vi "Methods_Insert Dividers.vi"(11 "Methods[] In":T1(array[cluster])) -> (3 "Methods[] Out":T1(array[cluster]))   [LabVIEW 2023] (continued)
Symbols:Set To Custom Symbol"}, "Method Flags"={"IsDeprecated"=FALSE, "IsPrivate"=FALSE, "IsScripting"=FALSE, "IsNotInRun-Time"=FALSE}, "Divider"=FALSE}, {"Class Info"={"Unique ID string"="66", "Parent ID string"="6", "Class Name (unlocalized)"="TreeControl", "Class Name (localized)"="TreeControl"}, "Method Info"={"Unique ID string"="756a3812", "Data name"="Custom Item Symbols.Set Symbol Array", "Short name (localized)"="Custom Item Symbols.Set Symbol Array", "Long name (localized)"="Custom Item Symbols:Set To Custom Symbol Array"}, "Method Flags"={"IsDeprecated"=FALSE, "IsPrivate"=FALSE, "IsScripting"=FALSE, "IsNotInRun-Time"=FALSE}, "Divider"=FALSE}, {"Class Info"={"Unique ID string"="66", "Parent ID string"="6", "Class Name (unlocalized)"="TreeControl", "Class Name (localized)"="TreeControl"}, "Method Info"={"Unique ID string"="756a3813", "Data name"="Custom Item Symbols.Revert Symbol", "Short name (localized)"="Custom Item Symbols.Revert Symbol", "Long name (localized)"="Custom Item Symbols:Revert To Built In Symbol"}, "Method Flags"={"IsDeprecated"=FALSE, "IsPrivate"=FALSE, "IsScripting"=FALSE, "IsNotInRun-Time"=FALSE}, "Divider"=FALSE}, {"Class Info"={"Unique ID string"="66", "Parent ID string"="6", "Class Name (unlocalized)"="TreeControl", "Class Name (localized)"="TreeControl"}, "Method Info"={"Unique ID string"="756a3814", "Data name"="Custom Item Symbols.Revert Symbols", "Short name (localized)"="Custom Item Symbols.Revert Symbols", "Long name (localized)"="Custom Item Symbols:Revert All To Built In Symbols"}, "Method Flags"={"IsDeprecated"=FALSE, "IsPrivate"=FALSE, "IsScripting"=FALSE, "IsNotInRun-Time"=FALSE}, "Divider"=FALSE}, {"Class Info"={"Unique ID string"="66", "Parent ID string"="6", "Class Name (unlocalized)"="TreeControl", "Class Name (localized)"="TreeControl"}, "Method Info"={"Unique ID string"="756a3815", "Data name"="Point To Row Column", "Short name (localized)"="Point To Row Column", "Long name (localized)"="Point to Row Column"}, "Method Flags"={"IsDeprecated"=FALSE, "IsPrivate"=FALSE, "IsScripting"=FALSE, "IsNotInRun-Time"=FALSE}, "Divider"=FALSE}, {"Class Info"={"Unique ID string"="66", "Parent ID string"="6", "Class Name (unlocalized)"="TreeControl", "Class Name (localized)"="TreeControl"}, "Method Info"={"Unique ID string"="756a3816", "Data name"="Navigate Tree.Get Previous", "Short name (localized)"="Navigate Tree.Get Previous", "Long name (localized)"="Navigate Tree:Get Previous Item"}, "Method Flags"={"IsDeprecated"=FALSE, "IsPrivate"=FALSE, "IsScripting"=FALSE, "IsNotInRun-Time"=FALSE}, "Divider"=FALSE}, {"Class Info"={"Unique ID string"="66", "Parent ID string"="6", "Class Name (unlocalized)"="TreeControl", "Class Name (localized)"="TreeControl"}, "Method Info"={"Unique ID string"="756a3817", "Data name"="Edit Tree Items.Add Multiple Items to End", "Short name (localized)"="Edit Tree Items.Add Multiple Items to End", "Long name (localized)"="Edit Tree Items:Add Multiple Items to End"}, "Method Flags"={"IsDeprecated"=FALSE, "IsPrivate"=FALSE, "IsScripting"=FALSE, "IsNotInRun-Time"=FALSE}, "Divider"=FALSE}, {"Class Info"={"Unique ID string"="71", "Parent ID string"="6", "Class Name (unlocalized)"="PlugInDDODummyContainer", "Class Name (localized)"="PlugInDDODummyContainer"}, "Method Info"={"Unique ID string"="47813c00", "Data name"="Dummy", "Short name (localized)"="Dummy", "Long name (localized)"="Dummy"}, "Method Flags"={"IsDeprecated"=FALSE, "IsPrivate"=TRUE, "IsScripting"=FALSE, "IsNotInRun-Time"=FALSE}, "Divider"=FALSE}, {"Class Info"={"Unique ID string"="73", "Parent ID string"="", "Class Name (unlocalized)"="Project", "Class Name (localized)"="Project"}, "Method Info"={"Unique ID string"="27109002", "Data name"="Close", "Short name (localized)"="Close", "Long name (localized)"="Close"}, "Method Flags"={"IsDeprecated"=FALSE, "IsPrivate"=FALSE, "IsScripting"=FALSE, "IsNotInRun-Time"=FALSE}, "Divider"=FALSE}, {"Class Info"={"Unique ID string"="73", "Parent ID string"="", "Class Name (unlocalized)"="Project", "Class Name (localized)"="Project"}, "Method Info"={"Unique ID string"="27109003", "Data name"="Save", "Short name (localized)"="Save", "Long name (localized)"="Save"}, "Method Flags"={"IsDeprecated"=FALSE, "IsPrivate"=FALSE, "IsScripting"=FALSE, "IsNotInRun-Time"=TRUE}, "Divider"=FALSE}, {"Class Info"={"Unique ID string"="73", "Parent ID string"="", "Class Name (unlocalized)"="Project", "Class Name (localized)"="Project"}, "Method Info"={"Unique ID string"="27109006", "Data name"="Item From Item ID", "Short name (localized)"="Item From Item ID", "Long name (localized)"="Item From Item ID"}, "Method Flags"={"IsDeprecated"=FALSE, "IsPrivate"=TRUE, "IsScripting"=FALSE, "IsNotInRun-Time"=TRUE}, "Divider"=FALSE}, {"Class Info"={"Unique ID string"="73", "Parent ID string"="", "Class Name (unlocalized)"="Project", "Class Name (localized)"="Project"}, "Method Info"={"Unique ID string"="27109009", "Data name"="Open Window", "Short name (localized)"="Open Window", "Long name (localized)"="Open Window"}, "Method Flags"={"IsDeprecated"=FALSE, "IsPrivate"=FALSE, "IsScripting"=FALSE, "IsNotInRun-Time"=TRUE}, "Divider"=FALSE}, {"Class Info"={"Unique ID string"="73", "Parent ID string"="", "Class Name (unlocalized)"="Project", "Class Name (localized)"="Project"}, "Method Info"={"Unique ID string"="2710900a", "Data name"="Close Window", "Short name (localized)"="Close Window", "Long name (localized)"="Close Window"}, "Method Flags"={"IsDeprecated"=FALSE, "IsPrivate"=FALSE, "IsScripting"=FALSE, "IsNotInRun-Time"=TRUE}, "Divider"=FALSE}, {"Class Info"={"Unique ID string"="73", "Parent ID string"="", "Class Name (unlocalized)"="Project", "Class Name (localized)"="Project"}, "Method Info"={"Unique ID string"="2710900c", "Data name"="Create Context For Type", "Short name (localized)"="Create Context For Type", "Long name (localized)"="Create Context For Type"}, "Method Flags"={"IsDeprecated"=FALSE, "IsPrivate"=TRUE, "IsScripting"=FALSE, "IsNotInRun-Time"=TRUE}, "Divider"=FALSE}, {"Class Info"={"Unique ID string"="73", "Parent ID string"="", "Class Name (unlocalized)"="Project", "Class Name (localized)"="Project"}, "Method Info"={"Unique ID string"="2710900d", "Data name"="Create Context For Instance", "Short name (localized)"="Create Context For Instance", "Long name (localized)"="Create Context For Instance"}, "Method Flags"={"IsDeprecated"=FALSE, "IsPrivate"=TRUE, "IsScripting"=FALSE, "IsNotInRun-Time"=TRUE}, "Divider"=FALSE}, {"Class Info"={"Unique ID string"="73", "Parent ID string"="", "Class Name (unlocalized)"="Project", "Class Name (localized)"="Project"}, "Method Info"={"Unique ID string"="27109012", "Data name"="Copy From Project", "Short name (localized)"="Copy From Project", "Long name (localized)"="Copy From Project"}, "Method Flags"={"IsDeprecated"=FALSE, "IsPrivate"=TRUE, "IsScripting"=FALSE, "IsNotInRun-Time"=TRUE}, "Divider"=FALSE}, {"Class Info"={"Unique ID string"="73", "Parent ID string"="", "Class Name (unlocalized)"="Project", "Class Name (localized)"="Project"}, "Method Info"={"Unique ID string"="27109013", "Data name"="Copy To Project", "Short name (localized)"="Copy To Project", "Long name (localized)"="Copy To Project"}, "Method Flags"={"IsDeprecated"=FALSE, "IsPrivate"=TRUE, "IsScripting"=FALSE, "IsNotInRun-Time"=TRUE}, "Divider"=FALSE}, {"Class Info"={"Unique ID string"="73", "Parent ID string"="", "Class Name (unlocalized)"="Project", "Class Name (localized)"="Project"}, "Method Info"={"Unique ID string"="27109014", "Data name"="Do Interactive Save", "Short name (localized)"="Do Interactive Save", "Long name (localized)"="Do Interactive Save"}, "Method Flags"={"IsDeprecated"=FALSE, "IsPrivate"=TRUE, "IsScripting"=FALSE, "IsNotInRun-Time"=TRUE}, "Divider"=FALSE}, {"Class Info"={"Unique ID string"="73", "Parent ID string"="", "Class Name (unlocalized)"="Project", "Class Name (localized)"="Project"}, "Method Info"={"Unique ID string"="27109015", "Data name"="Deploy Items", "Short name (localized)"="Deploy Items", "Long name (localized)"="Deploy Items"}, "Method Flags"={"IsDeprecated"=FALSE, "IsPrivate"=FALSE, "IsScripting"=FALSE, "IsNotInRun-Time"=TRUE}, "Divider"=FALSE}, {"Class Info"={"Unique ID string"="73", "Parent ID string"="", "Class Name (unlocalized)"="Project", "Class Name (localized)"="Project"}, "Method Info"={"Unique ID string"="27109016", "Data name"="Start Items", "Short name (localized)"="Start Items", "Long name (localized)"="Start Items"}, "Method Flags"={"IsDeprecated"=FALSE, "IsPrivate"=TRUE, "IsScripting"=FALSE, "IsNotInRun-Time"=TRUE}, "Divider"=FALSE}, {"Class Info"={"Unique ID string"="73", "Parent ID string"="", "Class Name (unlocalized)"="Project", "Class Name (localized)"="Project"}, "Method Info"={"Unique ID string"="27109017", "Data name"="Stop Items", "Short name (localized)"="Stop Items", "Long name (localized)"="Stop Items"}, "Method Flags"={"IsDeprecated"=FALSE, "IsPrivate"=TRUE, "IsScripting"=FALSE, "IsNotInRun-Time"=TRUE}, "Divider"=FALSE}, {"Class Info"={"Unique ID string"="73", "Parent ID string"="", "Class Name (unlocalized)"="Project", "Class Name (localized)"="Project"}, "Method Info"={"Unique ID string"="27109018", "Data name"="Undeploy Items", "Short name (localized)"="Undeploy Items", "Long name (localized)"="Undeploy Items"}, "Method Flags"={"IsDeprecated"=FALSE, "IsPrivate"=FALSE, "IsScripting"=FALSE, "IsNotInRun-Time"=TRUE}, "Divider"=FALSE}, {"Class Info"={"Unique ID string"="73", "Parent ID string"="", "Class Name (unlocalized)"="Project", "Class Name (localized)"="Project"}, "Method Info"={"Unique ID string"="2710901a", "Data name"="Save Specified Dirty Items", "Short name (localized)"="Save Specified Dirty Items", "Long name (localized)"="Save Specified Dirty Items"}, "Method Flags"={"IsDeprecated"=FALSE, "IsPrivate"=TRUE, "IsScripting"=FALSE, "IsNotInRun-Time"=TRUE}, "Divider"=FALSE}, {"Class Info"={"Unique ID string"="73", "Parent ID string"="", "Class Name (unlocalized)"="Project", "Class Name (localized)"="Project"}, "Method Info"={"Unique ID string"="2710901b", "Data name"="Proj Item From Ref", "Short name (localized)"="Proj Item From Ref", "Long name (localized)"="Get Project Item From VI Ref"}, "Method Flags"={"IsDeprecated"=FALSE, "IsPrivate"=TRUE, "IsScripting"=FALSE, "IsNotInRun-Time"=TRUE}, "Divider"=FALSE}, {"Class Info"={"Unique ID string"="73", "Parent ID string"="", "Class Name (unlocalized)"="Project", "Class Name (localized)"="Project"}, "Method Info"={"Unique ID string"="2710901c", "Data name"="PreviewDataFiles", "Short name (localized)"="PreviewDataFiles", "Long name (localized)"="Preview Data Files"}, "Method Flags"={"IsDeprecated"=FALSE, "IsPrivate"=TRUE, "IsScripting"=FALSE, "IsNotInRun-Time"=TRUE}, "Divider"=FALSE}, {"Class Info"={"Unique ID string"="73", "Parent ID string"="", "Class Name (unlocalized)"="Project", "Class Name (localized)"="Project"}, "Method Info"={"Unique ID string"="2710901e", "Data name"="Write Data Files", "Short name (localized)"="Write Data Files", "Long name (localized)"="Write Data Files"}, "Method Flags"={"IsDeprecated"=FALSE, "IsPrivate"=TRUE, "IsScripting"=FALSE, "IsNotInRun-Time"=TRUE}, "Divider"=FALSE}, {"Class Info"={"Unique ID string"="73", "Parent ID string"="", "Class Name (unlocalized)"="Project", "Class Name (localized)"="Project"}, "Method Info"={"Unique ID string"="2710901f", "Data name"="Get Bld Tokens", "Short name (localized)"="Get Bld Tokens", "Long name (localized)"="Get Build Tokens"}, "Method Flags"={"IsDeprecated"=FALSE, "IsPrivate"=TRUE, "IsScripting"=FALSE, "IsNotInRun-Time"=TRUE}, "Divider"=FALSE}, {"Class Info"={"Unique ID string"="73", "Parent ID string"="", "Class Name (unlocalized)"="Project", "Class Name (localized)"="Project"}, "Method Info"={"Unique ID string"="27109020", "Data name"="Query Type Behavior", "Short name (localized)"="Query Type Behavior", "Long name (localized)"="Query Type Behavior"}, "Method Flags"={"IsDeprecated"=FALSE, "IsPrivate"=TRUE, "IsScripting"=FALSE, "IsNotInRun-Time"=TRUE}, "Divider"=FALSE}, {"Class Info"={"Unique ID string"="73", "Parent ID string"="", "Class Name (unlocalized)"="Project", "Class Name (localized)"="Project"}, "Method Info"={"Unique ID string"="27109021", "Data name"="Open Application", "Short name (localized)"="Open Application", "Long name (localized)"="Open Application"}, "Method Flags"={"IsDeprecated"=FALSE, "IsPrivate"=TRUE, "IsScripting"=FALSE, "IsNotInRun-Time"=FALSE}, "Divider"=FALSE}, {"Class Info"={"Unique ID string"="73", "Parent ID string"="", "Class Name (unlocalized)"="Project", "Class Name (localized)"="Project"}, "Method Info"={"Unique ID string"="27109022", "Data name"="Has Behaviors", "Short name (localized)"="Has Behaviors", "Long name (localized)"="Has Behaviors"}, "Method Flags"={"IsDeprecated"=FALSE, "IsPrivate"=TRUE, "IsScripting"=FALSE, "IsNotInRun-Time"=TRUE}, "Divider"=FALSE}, {"Class Info"={"Unique ID string"="73", "Parent ID string"="", "Class Name (unlocalized)"="Project", "Class Name (localized)"="Project"}, "Method Info"={"Unique ID string"="27109023", "Data name"="Populate Provider Tree", "Short name (localized)"="Populate Provider Tree", "Long name (localized)"="Populate Provider Tree"}, "Method Flags"={"IsDeprecated"=FALSE, "IsPrivate"=TRUE, "IsScripting"=FALSE, "IsNotInRun-Time"=TRUE}, "Divider"=FALSE}, {"Class Info"={"Unique ID string"="73", "Parent ID string"="", "Class Name (unlocalized)"="Project", "Class Name (localized)"="Project"}, "Method Info"={"Unique ID string"="27109024", "Data name"="Save For Previous", "Short name (localized)"="Save For Previous", "Long name (localized)"="Save For Previous"}, "Method Flags"={"IsDeprecated"=FALSE, "IsPrivate"=FALSE, "IsScripting"=FALSE, "IsNotInRun-Time"=TRUE}, "Divider"=FALSE}, {"Class Info"={"Unique ID string"="73", "Parent ID string"="", "Class Name (unlocalized)"="Project", "Class Name (localized)"="Project"}, "Method Info"={"Unique ID string"="27109025", "Data name"="PostNoClose", "Short name (localized)"="PostNoClose", "Long name (localized)"="PostCloseLater"}, "Method Flags"={"IsDeprecated"=FALSE, "IsPrivate"=TRUE, "IsScripting"=TRUE, "IsNotInRun-Time"=TRUE}, "Divider"=FALSE}, {"Class Info"={"Unique ID string"="73", "Parent ID string"="", "Class Name (unlocalized)"="Project", "Class Name (localized)"="Project"}, "Method Info"={"Unique ID string"="27109026", "Data name"="Save As", "Short name (localized)"="Save As", "Long name (localized)"="Save As"}, "Method Flags"={"IsDeprecated"=FALSE, "IsPrivate"=FALSE, "IsScripting"=FALSE, "IsNotInRun-Time"=TRUE}, "Divider"=FALSE}, {"Class Info"={"Unique ID string"="73", "Parent ID string"="", "Class Name (unlocalized)"="Project", "Class Name (localized)"="Project"}, "Method Info"={"Unique ID string"="27109027", "Data name"="SaveCopy", "Short name (localized)"="SaveCopy", "Long name (localized)"="Save Copy"}, "Method Flags"={"IsDeprecated"=FALSE, "IsPrivate"=FALSE, "IsScripting"=FALSE, "IsNotInRun-Time"=TRUE}, "Divider"=FALSE}, {"Class Info"={"Unique ID string"="73", "Parent ID string"="", "Class Name (unlocalized)"="Project", "Class Name (localized)"="Project"}, "Method Info"={"Unique ID string"="27109028", "Data name"="Save Items for SCC", "Short name (localized)"="Save Items for SCC", "Long name (localized)"="Save Items for SCC"}, "Method Flags"={"IsDeprecated"=FALSE, "IsPrivate"=TRUE, "IsScripting"=FALSE, "IsNotInRun-Time"=TRUE}, "Divider"=FALSE}, {"Class Info"={"Unique ID string"="73", "Parent ID string"="", "Class Name (unlocalized)"="Project", "Class Name (localized)"="Project"}, "Method Info"={"Unique ID string"="27109029", "Data name"="MoveFiles", "Short name (localized)"="MoveFiles", "Long name (localized)"="MoveFiles"}, "Method Flags"={"IsDeprecated"=FALSE, "IsPrivate"=TRUE, "IsScripting"=FALSE, "IsNotInRun-Time"=FALSE}, "Divider"=FALSE}, {"Class Info"={"Unique ID string"="73", "Parent ID string"="", "Class Name (unlocalized)"="Project", "Class Name (localized)"="Project"}, "Method Info"={"Unique ID string"="2710902a", "Data name"="RenameFiles", "Short name (localized)"="RenameFiles", "Long name (localized)"="RenameFiles"}, "Method Flags"={"IsDeprecated"=FALSE, "IsPrivate"=TRUE, "IsScripting"=FALSE, "IsNotInRun-Time"=FALSE}, "Divider"=FALSE}, {"Class Info"={"Unique ID string"="73", "Parent ID string"="", "Class Name (unlocalized)"="Project", "Class Name (localized)"="Project"}, "Method Info"={"Unique ID string"="2710902b", "Data name"="RenameFilesDialogs", "Short name (localized)"="RenameFilesDialogs", "Long name (localized)"="RenameFilesDialogs"}, "Method Flags"={"IsDeprecated"=FALSE, "IsPrivate"=TRUE, "IsScripting"=FALSE, "IsNotInRun-Time"=FALSE}, "Divider"=FALSE}, {"Class Info"={"Unique ID string"="73", "Parent ID string"="", "Class Name (unlocalized)"="Project", "Class Name (localized)"="Project"}, "Method Info"={"Unique ID string"="2710902c", "Data name"="MoveFilesDialogs", "Short name (localized)"="MoveFilesDialogs", "Long name (localized)"="MoveFilesDialogs"}, "Method Flags"={"IsDeprecated"=FALSE, "IsPrivate"=TRUE, "IsScripting"=FALSE, "IsNotInRun-Time"=FALSE}, "Divider"=FALSE}, {"Class Info"={"Unique ID string"="73", "Parent ID string"="", "Class Name (unlocalized)"="Project", "Class Name (localized)"="Project"}, "Method Info"={"Unique ID string"="2710902d", "Data name"="MoveFolderContents", "Short name (localized)"="MoveFolderContents", "Long name (localized)"="MoveFolderContents"}, "Method Flags"={"IsDeprecated"=FALSE, "IsPrivate"=TRUE, "IsScripting"=FALSE, "IsNotInRun-Time"=FALSE}, "Divider"=FALSE}, {"Class Info"={"Unique ID string"="73", "Parent ID string"="", "Class Name (unlocalized)"="Project", "Class Name (localized)"="Project"}, "Method Info"={"Unique ID string"="2710902e", "Data name"="MoveFolderContentsDialog", "Short name (localized)"="MoveFolderContentsDialog", "Long name (localized)"="MoveFolderContentsDialog"}, "Method Flags"={"IsDeprecated"=FALSE, "IsPrivate"=TRUE, "IsScripting"=FALSE, "IsNotInRun-Time"=FALSE}, "Divider"=FALSE}, {"Class Info"={"Unique ID string"="73", "Parent ID string"="", "Class Name (unlocalized)"="Project", "Class Name (localized)"="Project"}, "Method Info"={"Unique ID string"="2710902f", "Data name"="Get Item", "Short name (localized)"="Get Item", "Long name (localized)"="Local Project Settings:Get Item"}, "Method Flags"={"IsDeprecated"=FALSE, "IsPrivate"=FALSE, "IsScripting"=FALSE, "IsNotInRun-Time"=FALSE}, "Divider"=FALSE}, {"Class Info"={"Unique ID string"="73", "Parent ID string"="", "Class Name (unlocalized)"="Project", "Class Name (localized)"="Project"}, "Method Info"={"Unique ID string"="27109030", "Data name"="Set Item", "Short name (localized)"="Set Item", "Long name (localized)"="Local Project Settings:Set Item"}, "Method Flags"={"IsDeprecated"=FALSE, "IsPrivate"=FALSE, "IsScripting"=FALSE, "IsNotInRun-Time"=TRUE}, "Divider"=FALSE}, {"Class Info"={"Unique ID string"="73", "Parent ID string"="", "Class Name (unlocalized)"="Project", "Class Name (localized)"="Project"}, "Method Info"={"Unique ID string"="27109031", "Data name"="Delete Item", "Short name (localized)"="Delete Item", "Long name (localized)"="Local Project Settings:Delete Item"}, "Method Flags"={"IsDeprecated"=FALSE, "IsPrivate"=FALSE, "IsScripting"=FALSE, "IsNotInRun-Time"=TRUE}, "Divider"=FALSE}, {"Class Info"={"Unique ID string"="73", "Parent ID string"="", "Class Name (unlocalized)"="Project", "Class Name (localized)"="Project"}, "Method Info"={"Unique ID string"="27109032", "Data name"="Delete Section", "Short name (localized)"="Delete Section", "Long name (localized)"="Local Project Settings:Delete Section"}, "Method Flags"={"IsDeprecated"=FALSE, "IsPrivate"=FALSE, "IsScripting"=FALSE, "IsNotInRun-Time"=TRUE}, "Divider"=FALSE}, {"Class Info"={"Unique ID string"="73", "Parent ID string"="", "Class Name (unlocalized)"="Project", "Class Name (localized)"="Project"}, "Method Info"={"Unique ID string"="27109033", "Data name"="Has Item", "Short name (localized)"="Has Item", "Long name (localized)"="Local Project Settings:Has Item"}, "Method Flags"={"IsDeprecated"=FALSE, "IsPrivate"=FALSE, "IsScripting"=FALSE, "IsNotInRun-Time"=FALSE}, "Divider"=FALSE}, {"Class Info"={"Unique ID string"="73", "Parent ID string"="", "Class Name (unlocalized)"="Project", "Class Name (localized)"="Project"}, "Method Info"={"Unique ID string"="27109034", "Data name"="Has Section", "Short name (localized)"="Has Section", "Long name (localized)"="Local Project Settings:Has Section"}, "Method Flags"={"IsDeprecated"=FALSE, "IsPrivate"=FALSE, "IsScripting"=FALSE, "IsNotInRun-Time"=FALSE}, "Divider"=FALSE}, {"Class Info"={"Unique ID string"="73", "Parent ID string"="", "Class Name (unlocalized)"="Project", "Class Name (localized)"="Project"}, "Method Info"={"Unique ID string"="27109035", "Data name"="SuppressChangeNotifications", "Short name (localized)"="SuppressChangeNotifications", "Long name (localized)"="SuppressChangeNotifications"}, "Method Flags"={"IsDeprecated"=FALSE, "IsPrivate"=TRUE, "IsScripting"=FALSE, "IsNotInRun-Time"=FALSE}, "Divider"=FALSE}, {"Class Info"={"Unique ID string"="73", "Parent ID string"="", "Class Name (unlocalized)"="Project", "Class Name (localized)"="Project"}, "Method Info"={"Unique ID string"="27109036", "Data name"="Save As Test", "Short name (localized)"="Save As Test", "Long name (localized)"="Save As Test"}, "Method Flags"={"IsDeprecated"=FALSE, "IsPrivate"=TRUE, "IsScripting"=FALSE, "IsNotInRun-Time"=FALSE}, "Divider"=FALSE}, {"Class Info"={"Unique ID string"="73", "Parent ID string"="", "Class Name (unlocalized)"="Project", "Class Name (localized)"="Project"}, "Method Info"={"Unique ID string"="27109037", "Data name"="IndustrialDeployItems", "Short name (localized)"="IndustrialDeployItems", "Long name (localized)"="Industrial Deploy Items"}, "Method Flags"={"IsDeprecated"=FALSE, "IsPrivate"=TRUE, "IsScripting"=FALSE, "IsNotInRun-Time"=FALSE}, "Divider"=FALSE}, {"Class Info"={"Unique ID string"="73", "Parent ID string"="", "Class Name (unlocalized)"="Project", "Class Name (localized)"="Project"}, "Method Info"={"Unique ID string"="27109038", "Data name"="BuildAssembliesFromProject", "Short name (localized)"="BuildAssembliesFromProject", "Long name (localized)"="Build Assemblies From Project"}, "Method Flags"={"IsDeprecated"=FALSE, "IsPrivate"=TRUE, "IsScripting"=FALSE, "IsNotInRun-Time"=TRUE}, "Divider"=FALSE}, {"Class Info"={"Unique ID string"="73", "Parent ID string"="", "Class Name (unlocalized)"="Project", "Class Name (localized)"="Project"}, "Method Info"={"Unique ID string"="27109039", "Data name"="ChangeCEMode", "Short name (localized)"="ChangeCEMode", "Long name (localized)"="Change Controller Engine Mode"}, "Method Flags"={"IsDeprecated"=FALSE, "IsPrivate"=TRUE, "IsScripting"=FALSE, "IsNotInRun-Time"=FALSE}, "Divider"=FALSE}, {"Class Info"={"Unique ID string"="73", "Parent ID string"="", "Class Name (unlocalized)"="Project", "Class Name (localized)"="Project"}, "Method Info"={"Unique ID string"="2710903a", "Data name"="GetItemsFromSourceID", "Short name (localized)"="GetItemsFromSourceID", "Long name (localized)"="Get Items From Source ID"}, "Method Flags"={"IsDeprecated"=FALSE, "IsPrivate"=TRUE, "IsScripting"=FALSE, "IsNotInRun-Time"=FALSE}, "Divider"=FALSE}, {"Class Info"={"Unique ID string"="73", "Parent ID string"="", "Class Name (unlocalized)"="Project", "Class Name (localized)"="Project"}, "Method Info"={"Unique ID string"="2710903b", "Data name"="BuildAssembliesToProject", "Short name (localized)"="BuildAssembliesToProject", "Long name (localized)"="Build Assemblies To Project"}, "Method Flags"={"IsDeprecated"=FALSE, "IsPrivate"=TRUE, "IsScripting"=FALSE, "IsNotInRun-Time"=TRUE}, "Divider"=FALSE}, {"Class Info"={"Unique ID string"="73", "Parent ID string"="", "Class Name (unlocalized)"="Project", "Class Name (localized)"="Project"}, "Method Info"={"Unique ID string"="2710903c", "Data name"="Set DocMod", "Short name (localized)"="Set DocMod", "Long name (localized)"="Set DocMod"}, "Method Flags"={"IsDeprecated"=FALSE, "IsPrivate"=TRUE, "IsScripting"=FALSE, "IsNotInRun-Time"=TRUE}, "Divider"=FALSE}, {"Class Info"={"Unique ID string"="73", "Parent ID string"="", "Class Name (unlocalized)"="Project", "Class Name (localized)"="Project"}, "Method Info"={"Unique ID string"="2710903d", "Data name"="DoQueuedNotifications", "Short name (localized)"="DoQueuedNotifications", "Long name (localized)"="DoQueuedNotifications"}, "Method Flags"={"IsDeprecated"=FALSE, "IsPrivate"=TRUE, "IsScripting"=FALSE, "IsNotInRun-Time"=FALSE}, "Divider"=FALSE}, {"Class Info"={"Unique ID string"="73", "Parent ID string"="", "Class Name (unlocalized)"="Project", "Class Name (localized)"="Project"}, "Method Info"={"Unique ID string"="2710903e", "Data name"="Refresh Auto-Populating Folders", "Short name (localized)"="Refresh Auto-Populating Folders", "Long name (localized)"="Refresh Auto-Populating Folders"}, "Method Flags"={"IsDeprecated"=FALSE, "IsPrivate"=FALSE, "IsScripting"=FALSE, "IsNotInRun-Time"=FALSE}, "Divider"=FALSE}, {"Class Info"={"Unique ID string"="73", "Parent ID string"="", "Class Name (unlocalized)"="Project", "Class Name (localized)"="Project"}, "Method Info"={"Unique ID string"="2710903f", "Data name"="Resolve Conflicts.Get Contents", "Short name (localized)"="Resolve Conflicts.Get Contents", "Long name (localized)"="Resolve Conflicts:Get Contents"}, "Method Flags"={"IsDeprecated"=FALSE, "IsPrivate"=TRUE, "IsScripting"=FALSE, "IsNotInRun-Time"=FALSE}, "Divider"=FALSE}, {"Class Info"={"Unique ID string"="73", "Parent ID string"="", "Class Name (unlocalized)"="Project", "Class Name (localized)"="Project"}, "Method Info"={"Unique ID string"="27109040", "Data name"="Resolve Conflicts.AutomateDlg", "Short name (localized)"="Resolve Conflicts.AutomateDlg", "Long name (localized)"="Resolve Conflicts:AutomateDlg"}, "Method Flags"={"IsDeprecated"=FALSE, "IsPrivate"=TRUE, "IsScripting"=FALSE, "IsNotInRun-Time"=FALSE}, "Divider"=FALSE}, {"Class Info"={"Unique ID string"="73", "Parent ID string"="", "Class Name (unlocalized)"="Project", "Class Name (localized)"="Project"}, "Method Info"={"Unique ID string"="27109041", "Data name"="Resolve Conflicts.UseSelectedItem", "Short name (localized)"="Resolve Conflicts.UseSelectedItem", "Long name (localized)"="Resolve Conflicts:UseSelectedItem"}, "Method Flags"={"IsDeprecated"=FALSE, "IsPrivate"=TRUE, "IsScripting"=FALSE, "IsNotInRun-Time"=FALSE}, "Divider"=FALSE}, {"Class Info"={"Unique ID string"="73", "Parent ID string"="", "Class Name (unlocalized)"="Project", "Class Name (localized)"="Project"}, "Method Info"={"Unique ID string"="27109042", "Data name"="Files View.Get Contents", "Short name (localized)"="Files View.Get Contents", "Long name (localized)"="Files View:Get Contents"}, "Method Flags"={"IsDeprecated"=FALSE, "IsPrivate"=TRUE, "IsScripting"=FALSE, "IsNotInRun-Time"=FALSE}, "Divider"=FALSE}, {"Class Info"={"Unique ID string"="73", "Parent ID string"="", "Class Name (unlocalized)"="Project", "Class Name (localized)"="Project"}, "Method Info"={"Unique ID string"="27109043", "Data name"="IndustrialUndeployAll", "Short name (localized)"="IndustrialUndeployAll", "Long name (localized)"="IndustrialUndeployAll"}, "Method Flags"={"IsDeprecated"=FALSE, "IsPrivate"=TRUE, "IsScripting"=FALSE, "IsNotInRun-Time"=FALSE}, "Divider"=FALSE}, {"Class Info"={"Unique ID string"="73", "Parent ID string"="", "Class Name (unlocalized)"="Project", "Class Name (localized)"="Project"}, "Method Info"={"Unique ID string"="27109044", "Data name"="IndustrialUndeployItems", "Short name (localized)"="IndustrialUndeployItems", "Long name (localized)"="IndustrialUndeployItems"}, "Method Flags"={"IsDeprecated"=FALSE, "IsPrivate"=TRUE, "IsScripting"=FALSE, "IsNotInRun-Time"=FALSE}, "Divider"=FALSE}, {"Class Info"={"Unique ID string"="73", "Parent ID string"="", "Class Name (unlocalized)"="Project", "Class Name (localized)"="Project"}, "Method Info"={"Unique ID string"="27109045", "Data name"="BeginIOScanTimeCollection", "Short name (localized)"="BeginIOScanTimeCollection", "Long name (localized)"="BeginIOScanTimeCollection"}, "Method Flags"={"IsDeprecated"=FALSE, "IsPrivate"=TRUE, "IsScripting"=FALSE, "IsNotInRun-Time"=TRUE}, "Divider"=FALSE}, {"Class Info"={"Unique ID string"="73", "Parent ID string"="", "Class Name (unlocalized)"="Project", "Class Name (localized)"="Project"}, "Method Info"={"Unique ID string"="27109046", "Data name"="EndIOScanCollection", "Short name (localized)"="EndIOScanCollection", "Long name (localized)"="EndIOScanCollection"}, "Method Flags"={"IsDeprecated"=FALSE, "IsPrivate"=TRUE, "IsScripting"=FALSE, "IsNotInRun-Time"=TRUE}, "Divider"=FALSE}, {"Class Info"={"Unique ID string"="73", "Parent ID string"="", "Class Name (unlocalized)"="Project", "Class Name (localized)"="Project"}, "Method Info"={"Unique ID string"="27109047", "Data name"="GetIOScanTime", "Short name (localized)"="GetIOScanTime", "Long name (localized)"="GetIOScanTime"}, "Method Flags"={"IsDeprecated"=FALSE, "IsPrivate"=TRUE, "IsScripting"=FALSE, "IsNotInRun-Time"=TRUE}, "Divider"=FALSE}, {"Class Info"={"Unique ID string"="73", "Parent ID string"="", "Class Name (unlocalized)"="Project", "Class Name (localized)"="Project"}, "Method Info"={"Unique ID string"="27109048", "Data name"="Create Context For Instance Without Sublib Loading", "Short name (localized)"="Create Context For Instance Without Sublib Loading", "Long name (localized)"="Create Context For Instance Without Sublib Loading"}, "Method Flags"={"IsDeprecated"=FALSE, "IsPrivate"=TRUE, "IsScripting"=FALSE, "IsNotInRun-Time"=TRUE}, "Divider"=FALSE}, {"Class Info"={"Unique ID string"="73", "Parent ID string"="", "Class Name (unlocalized)"="Project", "Class Name (localized)"="Project"}, "Method Info"={"Unique ID string"="27109049", "Data name"="Bounds", "Short name (localized)"="Bounds", "Long name (localized)"="Bounds"}, "Method Flags"={"IsDeprecated"=FALSE, "IsPrivate"=TRUE, "IsScripting"=FALSE, "IsNotInRun-Time"=FALSE}, "Divider"=FALSE}, {"Class Info"={"Unique ID string"="73", "Parent ID string"="", "Class Name (unlocalized)"="Project", "Class Name (localized)"="Project"}, "Method Info"={"Unique ID string"="2710904a", "Data name"="AutoDiscoverSupportsType", "Short name (localized)"="AutoDiscoverSupportsType", "Long name (localized)"="AutoDiscoverSupportsType"}, "Method Flags"={"IsDeprecated"=FALSE, "IsPrivate"=TRUE, "IsScripting"=FALSE, "IsNotInRun-Time"=FALSE}, "Divider"=FALSE}, {"Class Info"={"Unique ID string"="73", "Parent ID string"="", "Class Name (unlocalized)"="Project", "Class Name (localized)"="Project"}, "Method Info"={"Unique ID string"="2710904b", "Data name"="AutoDiscoverOverrideType", "Short name (localized)"="AutoDiscoverOverrideType", "Long name (localized)"="AutoDiscoverOverrideType"}, "Method Flags"={"IsDeprecated"=FALSE, "IsPrivate"=TRUE, "IsScripting"=FALSE, "IsNotInRun-Time"=FALSE}, "Divider"=FALSE}, {"Class Info"={"Unique ID string"="73", "Parent ID string"="", "Class Name (unlocalized)"="Project", "Class Name (localized)"="Project"}, "Method Info"={"Unique ID string"="2710904c", "Data name"="AutoDiscoverCallOverride", "Short name (localized)"="AutoDiscoverCallOverride", "Long name (localized)"="AutoDiscoverCallOverride"}, "Method Flags"={"IsDeprecated"=FALSE, "IsPrivate"=TRUE, "IsScripting"=FALSE, "IsNotInRun-Time"=FALSE}, "Divider"=FALSE}, {"Class Info"={"Unique ID string"="73", "Parent ID string"="", "Class Name (unlocalized)"="Project", "Class Name (localized)"="Project"}, "Method Info"={"Unique ID string"="2710904d", "Data name"="Populate Provider Tree Files View", "Short name (localized)"="Populate Provider Tree Files View", "Long name (localized)"="Populate Provider Tree (Files View)"}, "Method Flags"={"IsDeprecated"=FALSE, "IsPrivate"=TRUE, "IsScripting"=FALSE, "IsNotInRun-Time"=TRUE}, "Divider"=FALSE}, {"Class Info"={"Unique ID string"="73", "Parent ID string"="", "Class Name (unlocalized)"="Project", "Class Name (localized)"="Project"}, "Method Info"={"Unique ID string"="2710904e", "Data name"="GetFilesViewItem", "Short name (localized)"="GetFilesViewItem", "Long name (localized)"="GetFilesViewItem"}, "Method Flags"={"IsDeprecated"=FALSE, "IsPrivate"=TRUE, "IsScripting"=FALSE, "IsNotInRun-Time"=FALSE}, "Divider"=FALSE}, {"Class Info"={"Unique ID string"="73", "Parent ID string"="", "Class Name (unlocalized)"="Project", "Class Name (localized)"="Project"}, "Method Info"={"Unique ID string"="2710904f", "Data name"="UpdateFilesViewData", "Short name (localized)"="UpdateFilesViewData", "Long name (localized)"="UpdateFilesViewData"}, "Method Flags"={"IsDeprecated"=FALSE, "IsPrivate"=TRUE, "IsScripting"=FALSE, "IsNotInRun-Time"=FALSE}, "Divider"=FALSE}, {"Class Info"={"Unique ID string"="73", "Parent ID string"="", "Class Name (unlocalized)"="Project", "Class Name (localized)"="Project"}, "Method Info"={"Unique ID string"="27109050", "Data name"="Get Deployable Deps", "Short name (localized)"="Get Deployable Deps", "Long name (localized)"="Get Deployable Dependencies"}, "Method Flags"={"IsDeprecated"=FALSE, "IsPrivate"=TRUE, "IsScripting"=FALSE, "IsNotInRun-Time"=TRUE}, "Divider"=FALSE}, {"Class Info"={"Unique ID string"="73", "Parent ID string"="", "Class Name (unlocalized)"="Project", "Class Name (localized)"="Project"}, "Method Info"={"Unique ID string"="27109051", "Data name"="BrowseVariableDialog", "Short name (localized)"="BrowseVariableDialog", "Long name (localized)"="Browse Variable Dialog"}, "Method Flags"={"IsDeprecated"=FALSE, "IsPrivate"=FALSE, "IsScripting"=FALSE, "IsNotInRun-Time"=TRUE}, "Divider"=FALSE}, {"Class Info"={"Unique ID string"="73", "Parent ID string"="", "Class Name (unlocalized)"="Project", "Class Name (localized)"="Project"}, "Method Info"={"Unique ID string"="27109052", "Data name"="IsItemIDUnderDependencies", "Short name (localized)"="IsItemIDUnderDependencies", "Long name (localized)"="IsItemIDUnderDependencies"}, "Method Flags"={"IsDeprecated"=FALSE, "IsPrivate"=TRUE, "IsScripting"=FALSE, "IsNotInRun-Time"=FALSE}, "Divider"=FALSE}, {"Class Info"={"Unique ID string"="73", "Parent ID string"="", "Class Name (unlocalized)"="Project", "Class Name (localized)"="Project"}, "Method Info"={"Unique ID string"="27109053", "Data name"="Save As With Rename", "Short name (localized)"="Save As With Rename", "Long name (localized)"="Save As With Rename"}, "Method Flags"={"IsDeprecated"=FALSE, "IsPrivate"=TRUE, "IsScripting"=FALSE, "IsNotInRun-Time"=TRUE}, "Divider"=FALSE}, {"Class Info"={"Unique ID string"="73", "Parent ID string"="", "Class Name (unlocalized)"="Project", "Class Name (localized)"="Project"}, "Method Info"={"Unique ID string"="27109054", "Data name"="Save As With Rename Prog Inc", "Short name (localized)"="Save As With Rename Prog Inc", "Long name (localized)"="Save As With Rename Progress Increment"}, "Method Flags"={"IsDeprecated"=FALSE, "IsPrivate"=TRUE, "IsScripting"=FALSE, "IsNotInRun-Time"=TRUE}, "Divider"=FALSE}, {"Class Info"={"Unique ID string"="73", "Parent ID string"="", "Class Name (unlocalized)"="Project", "Class Name (localized)"="Project"}, "Method Info"={"Unique ID string"="27109055", "Data name"="Save As With Rename Prog Close", "Short name (localized)"="Save As With Rename Prog Close", "Long name (localized)"="Save As With Rename Progress Close"}, "Method Flags"={"IsDeprecated"=FALSE, "IsPrivate"=TRUE, "IsScripting"=FALSE, "IsNotInRun-Time"=TRUE}, "Divider"=FALSE}, {"Class Info"={"Unique ID string"="74", "Parent ID string"="", "Class Name (unlocalized)"="ProjectItem", "Class Name (localized)"="ProjectItem"}, "Method Info"={"Unique ID string"="35b53800", "Data name"="AddFile", "Short name (localized)"="AddFile", "Long name (localized)"="Add File"}, "Method Flags"={"IsDeprecated"=FALSE, "IsPrivate"=FALSE, "IsScripting"=FALSE, "IsNotInRun-Time"=TRUE}, "Divider"=FALSE}, {"Class Info"={"Unique ID string"="74", "Parent ID string"="", "Class Name (unlocalized)"="ProjectItem", "Class Name (localized)"="ProjectItem"}, "Method Info"={"Unique ID string"="35b53801", "Data name"="AddItem", "Short name (localized)"="AddItem", "Long name (localized)"="Add Item"}, "Method Flags"={"IsDeprecated"=FALSE, "IsPrivate"=FALSE, "IsScripting"=FALSE, "IsNotInRun-Time"=TRUE}, "Divider"=FALSE}, {"Class Info"={"Unique ID string"="74", "Parent ID string"="", "Class Name (unlocalized)"="ProjectItem", "Class Name (localized)"="ProjectItem"}, "Method Info"={"Unique ID string"="35b53803", "Data name"="Delete", "Short name (localized)"="Delete", "Long name (localized)"="Delete"}, "Method Flags"={"IsDeprecated"=FALSE, "IsPrivate"=FALSE, "IsScripting"=FALSE, "IsNotInRun-Time"=TRUE}, "Divider"=FALSE}, {"Class Info"={"Unique ID string"="74", "Parent ID string"="", "Class Name (unlocalized)"="ProjectItem", "Class Name (localized)"="ProjectItem"}, "Method Info"={"Unique ID string"="35b53809", "Data name"="CloseRefee", "Short name (localized)"="CloseRefee", "Long name (localized)"="Close Refee"}, "Method Flags"={"IsDeprecated"=FALSE, "IsPrivate"=TRUE, "IsScripting"=FALSE, "IsNotInRun-Time"=TRUE}, "Divider"=FALSE}, {"Class Info"={"Unique ID string"="74", "Parent ID string"="", "Class Name (unlocalized)"="ProjectItem", "Class Name (localized)"="ProjectItem"}, "Method Info"={"Unique ID string"="35b5380a", "Data name"="Debug Bind To Item", "Short name (localized)"="Debug Bind To Item", "Long name (localized)"="Debug Bind:To Item"}, "Method Flags"={"IsDeprecated"=FALSE, "IsPrivate"=TRUE, "IsScripting"=FALSE, "IsNotInRun-Time"=TRUE}, "Divider"=FALSE}, {"Class Info"={"Unique ID string"="74", "Parent ID string"="", "Class Name (unlocalized)"="ProjectItem", "Class Name (localized)"="ProjectItem"}, "Method Info"={"Unique ID string"="35b5380b", "Data name"="Debug Bind To Children", "Short name (localized)"="Debug Bind To Children", "Long name (localized)"="Debug Bind:To Children"}, "Method Flags"={"IsDeprecated"=FALSE, "IsPrivate"=TRUE, "IsScripting"=FALSE, "IsNotInRun-Time"=TRUE}, "Divider"=FALSE}, {"Class Info"={"Unique ID string"="74", "Parent ID string"="", "Class Name (unlocalized)"="ProjectItem", "Class Name (localized)"="ProjectItem"}, "Method Info"={"Unique ID string"="35b5380c", "Data name"="Get Tag", "Short name (localized)"="Get Tag", "Long name (localized)"="Tag:Get Tag"}, "Method Flags"={"IsDeprecated"=FALSE, "IsPrivate"=FALSE, "IsScripting"=FALSE, "IsNotInRun-Time"=FALSE}, "Divider"=FALSE}, {"Class Info"={"Unique ID string"="74", "Parent ID string"="", "Class Name (unlocalized)"="ProjectItem", "Class Name (localized)"="ProjectItem"}, "Method Info"={"Unique ID string"="35b5380d", "Data name"="Set Tag", "Short name (localized)"="Set Tag", "Long name (localized)"="Tag:Set Tag"}, "Method Flags"={"IsDeprecated"=FALSE, "IsPrivate"=FALSE, "IsScripting"=FALSE, "IsNotInRun-Time"=TRUE}, "Divider"=FALSE}, {"Class Info"={"Unique ID string"="74", "Parent ID string"="", "Class Name (unlocalized)"="ProjectItem", "Class Name (localized)"="ProjectItem"}, "Method Info"={"Unique ID string"="35b5380e", "Data name"="Delete Tag", "Short name (localized)"="Delete Tag", "Long name (localized)"="Tag:Delete"}, "Method Flags"={"IsDeprecated"=FALSE, "IsPrivate"=FALSE, "IsScripting"=FALSE, "IsNotInRun-Time"=TRUE}, "Divider"=FALSE}, {"Class Info"={"Unique ID string"="74", "Parent ID string"="", "Class Name (unlocalized)"="ProjectItem", "Class Name (localized)"="ProjectItem"}, "Method Info"={"Unique ID string"="35b5380f", "Data name"="Get Tag Names", "Short name (localized)"="Get Tag Names", "Long name (localized)"="Tag:Get Names"}, "Method Flags"={"IsDeprecated"=FALSE, "IsPrivate"=FALSE, "IsScripting"=FALSE, "IsNotInRun-Time"=FALSE}, "Divider"=FALSE}, {"Class Info"={"Unique ID string"="74", "Parent ID string"="", "Class Name (unlocalized)"="ProjectItem", "Class Name (localized)"="ProjectItem"}, "Method Info"={"Unique ID string"="35b53810", "Data name"="Get All Descendents", "Short name (localized)"="Get All Descendents", "Long name (localized)"="Get All Descendents"}, "Method Flags"={"IsDeprecated"=FALSE, "IsPrivate"=FALSE, "IsScripting"=FALSE, "IsNotInRun-Time"=FALSE}
